vi "Dispensaor de Snacks.vi"() -> ()   [LabVIEW 2021]
panel:
  in  "Ring":u16(ring)
  out "Enum":T1(ring)
  in  "Dinero":i16
  in  "Tab Control":enum32{"Dispensador", "Inventario"}(tab)
  in  "Panel Frontal":T2
  in  "Reset":bool
  in  "Dispensador":bool
  in  "Productos":T3
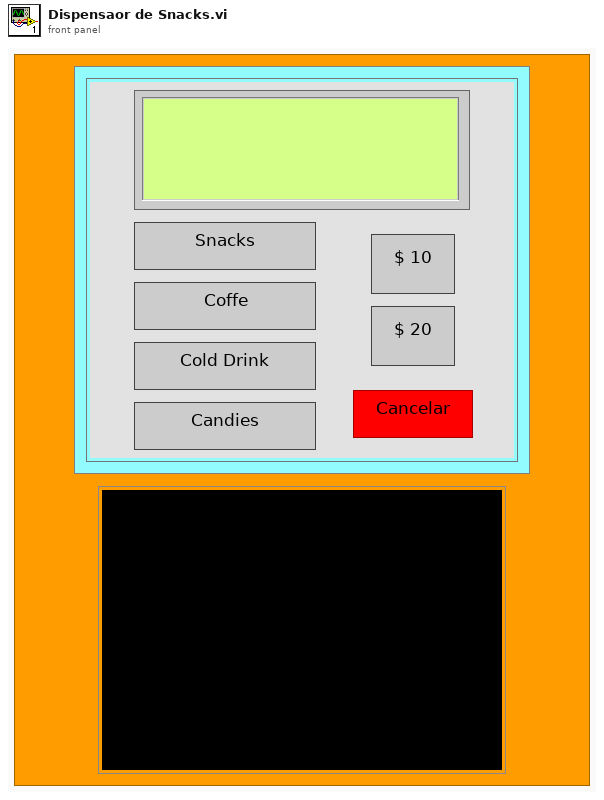
[diagram p1: front panel]
types:
  T1 = enum16{"Sin elegir", "Snacks", "Coffe", "Cold drink", "Candies"}
  T2 = cluster{"Snacks":bool, "Coffe":bool, "Cold drink":bool, "Candies":bool, "$ 10":bool, "$ 20":bool, "Cancelar":bool, "Pantalla":string, "Inventario":bool}
  T3 = cluster{"Snacks":i16, "Coffe":i16, "Cold drink":i16, "Candies":i16}
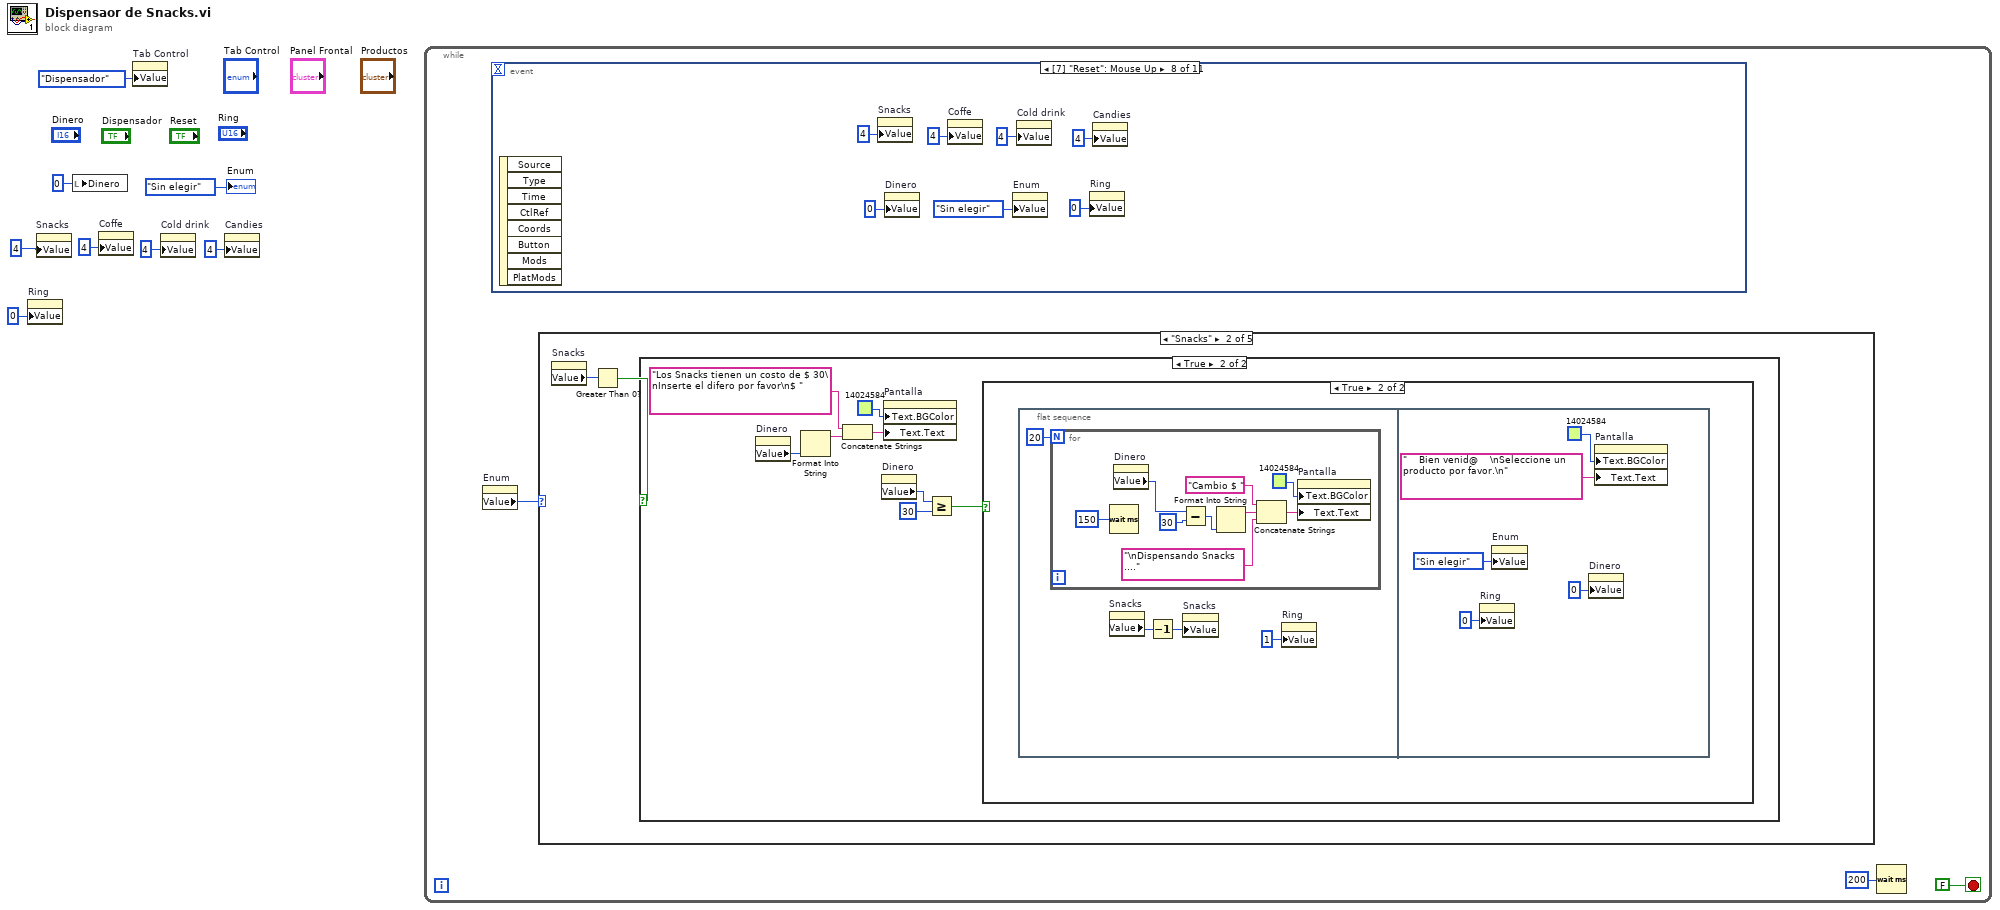
[diagram p0: block diagram]
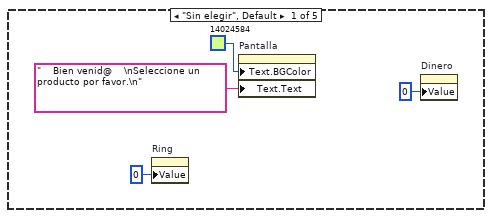
[diagram p2: hidden frame]
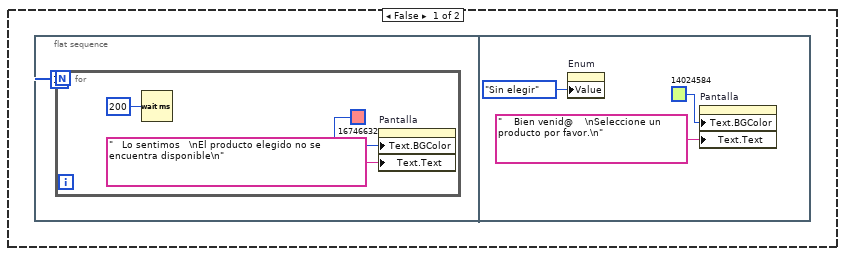
[diagram p3: hidden frame]
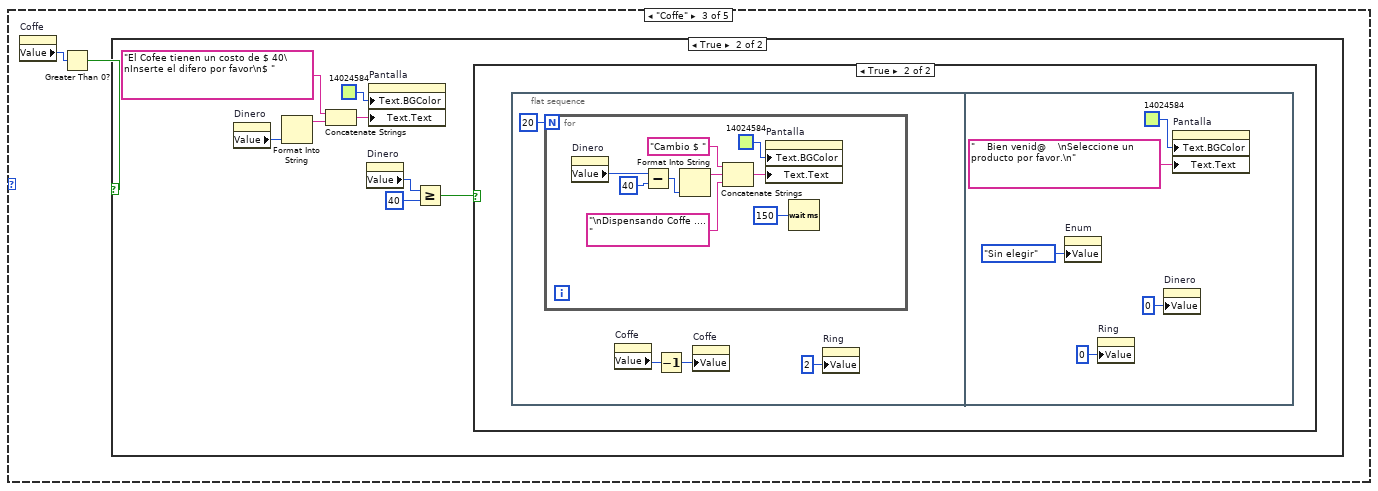
[diagram p5: hidden frame]
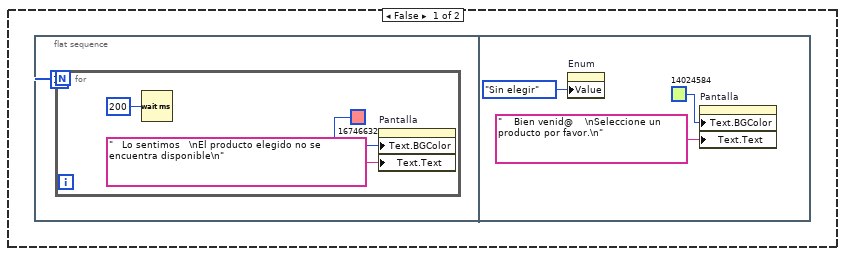
[diagram p6: hidden frame]
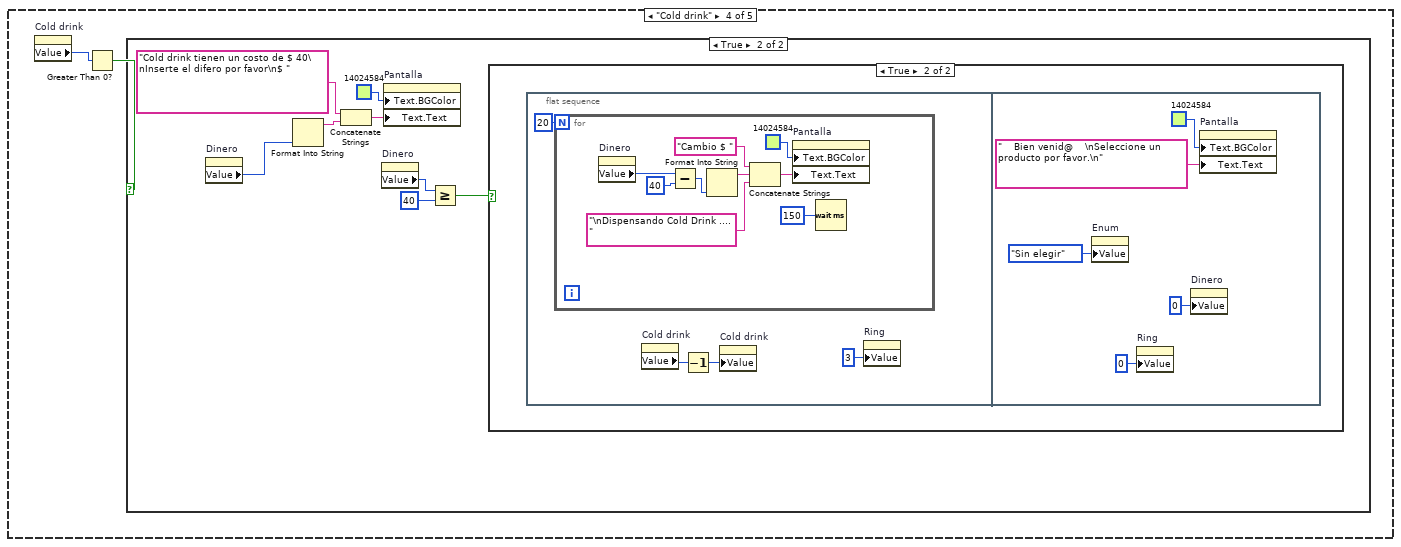
[diagram p8: hidden frame]
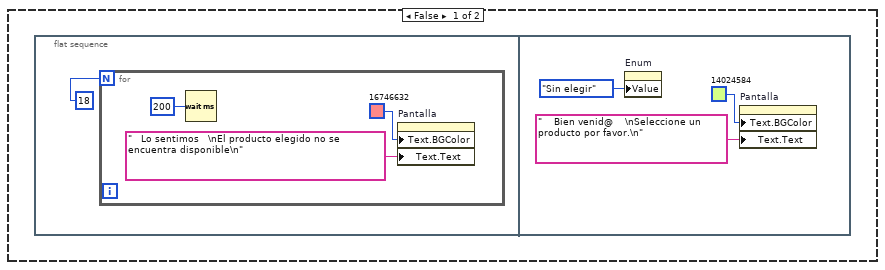
[diagram p9: hidden frame]
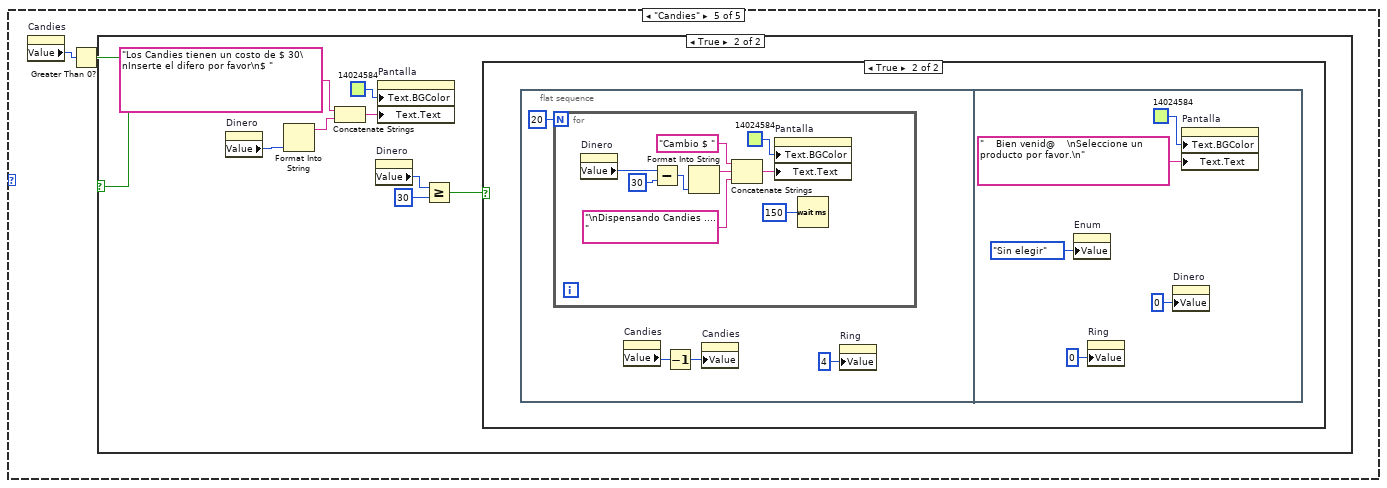
[diagram p11: hidden frame]
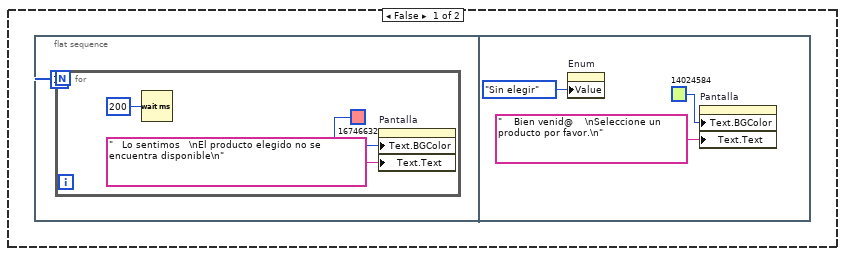
[diagram p12: hidden frame]
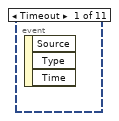
[diagram p14: hidden frame]
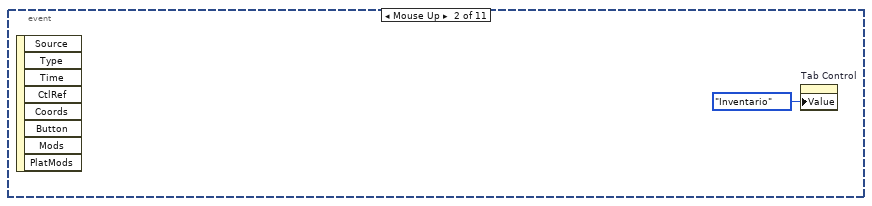
[diagram p15: hidden frame]
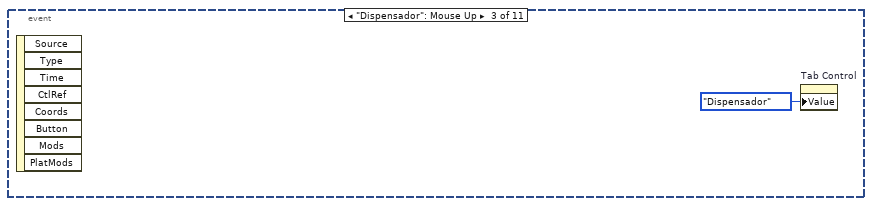
[diagram p16: hidden frame]
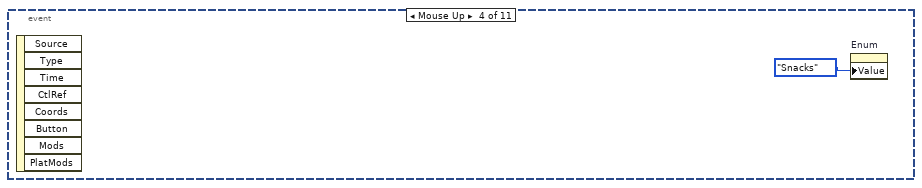
[diagram p17: hidden frame]
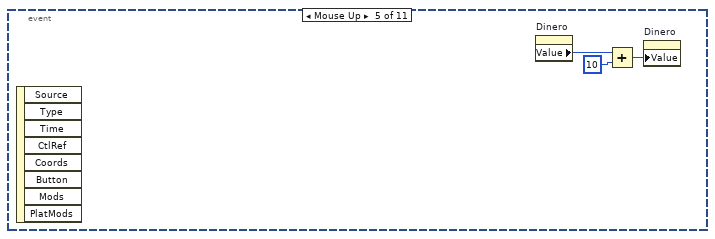
[diagram p18: hidden frame]
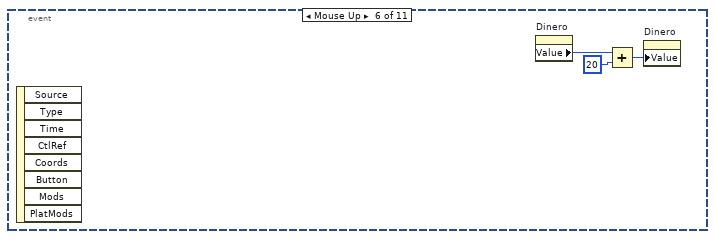
[diagram p19: hidden frame]
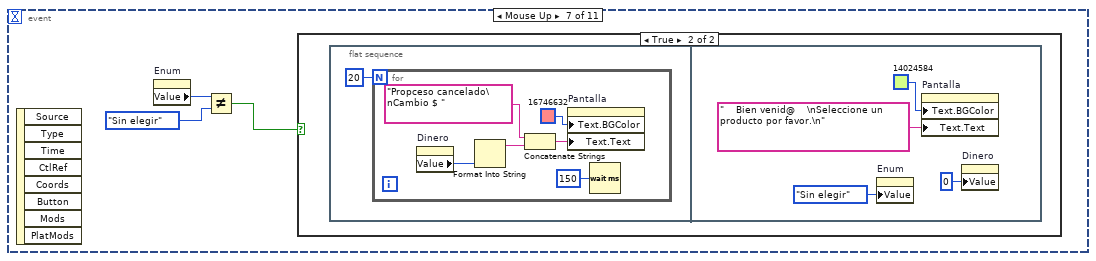
[diagram p20: hidden frame]
diagram:
  n1 = property on="Ring" class="Ring (strict)"("Value"=u16 0 ("Ring")) -> ()  [unwired: 2 in, 2 out]
  n2 = property on="Snacks" class="DigNum (strict)"("Value"=i16 4) -> ()  [unwired: 2 in, 2 out]
  n3 = local write "Dinero"(i16 0 ("Dinero")) -> ()
  n4 = property on="Coffe" class="DigNum (strict)"("Value"=i16 4) -> ()  [unwired: 2 in, 2 out]
  n5 = property on="Tab Control" class="TabCtl (strict)"("Value"=enum32{"Dispensador", "Inventario"}."Dispensador" ("Tab Control")) -> ()  [unwired: 2 in, 2 out]
  n6 = property on="Cold drink" class="DigNum (strict)"("Value"=i16 4) -> ()  [unwired: 2 in, 2 out]
  n7 = property on="Candies" class="DigNum (strict)"("Value"=i16 4) -> ()  [unwired: 2 in, 2 out]
  n8 = while {
    stop <- FALSE stop-if-true
    n9 = property on="Enum" class="Enum (strict)"() -> ("Value"=w9:T1)  [unwired: 2 in, 2 out]
    n10 = event shown="[7] \"Reset\": Mouse Up" {
      selector: _ -> [_ _ _ _ _ _ _ _ _ _ _]
      dyn-events: _ -> [_ _ _ _ _ _ _ _ _ _ _]
      timeout: _ -> [_ _ _ _ _ _ _ _ _ _ _]
      event Timeout {
        n11 = event-data() -> ()  [unwired: 1 in, 3 out]
      }
      event "Panel Frontal.Inventario": Mouse Up {
        n12 = event-data() -> ()  [unwired: 1 in, 8 out]
        n13 = property on="Tab Control" class="TabCtl (strict)"("Value"=enum32{"Dispensador", "Inventario"}."Inventario" ("Tab Control")) -> ()  [unwired: 2 in, 2 out]
      }
      event "Dispensador": Mouse Up {
        n14 = event-data() -> ()  [unwired: 1 in, 8 out]
        n15 = property on="Tab Control" class="TabCtl (strict)"("Value"=enum32{"Dispensador", "Inventario"}."Dispensador" ("Tab Control")) -> ()  [unwired: 2 in, 2 out]
      }
      event "Panel Frontal.Snacks": Mouse Up {
        n16 = event-data() -> ()  [unwired: 1 in, 8 out]
        n17 = property on="Enum" class="Enum (strict)"("Value"=T1."Snacks" ("Enum")) -> ()  [unwired: 2 in, 2 out]
      }
      event "Panel Frontal.$ 10": Mouse Up {
        n18 = event-data() -> ()  [unwired: 1 in, 8 out]
        n19 = property on="Dinero" class="DigNum (strict)"() -> ("Value"=w161:i16)  [unwired: 2 in, 2 out]
        n20 = Add(x=w161, y=i16 10) -> (x+y=w159:i16)
        n21 = property on="Dinero" class="DigNum (strict)"("Value"=w159) -> ()  [unwired: 2 in, 2 out]
      }
      event "Panel Frontal.$ 20": Mouse Up {
        n22 = event-data() -> ()  [unwired: 1 in, 8 out]
        n23 = property on="Dinero" class="DigNum (strict)"() -> ("Value"=w164:i16)  [unwired: 2 in, 2 out]
        n24 = Add(x=w164, y=i16 20) -> (x+y=w162:i16)
        n25 = property on="Dinero" class="DigNum (strict)"("Value"=w162) -> ()  [unwired: 2 in, 2 out]
      }
      event "Panel Frontal.Cancelar": Mouse Up {
        n26 = event-data() -> ()  [unwired: 1 in, 8 out]
        n27 = property on="Enum" class="Enum (strict)"() -> ("Value"=w167:T1)  [unwired: 2 in, 2 out]
        n28 = Not Equal?(x=w167, y=T1."Sin elegir") -> (x != y?=w165:bool)
        n29 = case shown="True" w165 {
          frame False {
          }
          frame True {
            n30 = flat-sequence {
              frame #0 {
                n31 = for {
                  N: 20 -> [_]
                  n32 = property on="Dinero" class="DigNum (strict)"() -> ("Value"=w173:i16)  [unwired: 2 in, 2 out]
                  n33 = Format Into String(w173) -> (resulting string=w171:string)  [unwired: 3 in, 1 out]
                  n34 = Concatenate Strings("Propceso cancelado\nCambio $ " ("Text.Text"), w171) -> (w170:string)
                  n35 = property on="Pantalla" class="Str"("Text.BGColor"=u32 16746632 ("Text.Text Colors:BG Color"), "Text.Text"=w170) -> ()  [unwired: 2 in, 2 out]
                  n36 = Wait (ms)(milliseconds to wait=u32 150) -> ()  [unwired: 1 out]
                }
              }
              frame #1 {
                n37 = property on="Enum" class="Enum (strict)"("Value"=T1."Sin elegir" ("Enum")) -> ()  [unwired: 2 in, 2 out]
                n38 = property on="Pantalla" class="Str"("Text.BGColor"=u32 14024584 ("Text.Text Colors:BG Color"), "Text.Text"="　 Bien venid@ 　\nSeleccione un producto por favor.\n") -> ()  [unwired: 2 in, 2 out]
                n39 = property on="Dinero" class="DigNum (strict)"("Value"=i16 0 ("Dinero")) -> ()  [unwired: 2 in, 2 out]
              }
            }
          }
        }
      }
      event "Reset": Mouse Up {
        n40 = event-data() -> ()  [unwired: 1 in, 8 out]
        n41 = property on="Snacks" class="DigNum (strict)"("Value"=i16 4) -> ()  [unwired: 2 in, 2 out]
        n42 = property on="Dinero" class="DigNum (strict)"("Value"=i16 0 ("Dinero")) -> ()  [unwired: 2 in, 2 out]
        n43 = property on="Coffe" class="DigNum (strict)"("Value"=i16 4) -> ()  [unwired: 2 in, 2 out]
        n44 = property on="Enum" class="Enum (strict)"("Value"=T1."Sin elegir" ("Enum")) -> ()  [unwired: 2 in, 2 out]
        n45 = property on="Cold drink" class="DigNum (strict)"("Value"=i16 4) -> ()  [unwired: 2 in, 2 out]
        n46 = property on="Ring" class="Ring (strict)"("Value"=u16 0 ("Ring")) -> ()  [unwired: 2 in, 2 out]
        n47 = property on="Candies" class="DigNum (strict)"("Value"=i16 4) -> ()  [unwired: 2 in, 2 out]
      }
      event "Panel Frontal.Cold drink": Mouse Up {
        n48 = event-data() -> ()  [unwired: 1 in, 8 out]
        n49 = property on="Enum" class="Enum (strict)"("Value"=T1."Cold drink" ("Enum")) -> ()  [unwired: 2 in, 2 out]
      }
      event "Panel Frontal.Candies": Mouse Up {
        n50 = event-data() -> ()  [unwired: 1 in, 8 out]
        n51 = property on="Enum" class="Enum (strict)"("Value"=T1."Candies" ("Enum")) -> ()  [unwired: 2 in, 2 out]
      }
      event "Panel Frontal.Coffe": Mouse Up {
        n52 = event-data() -> ()  [unwired: 1 in, 8 out]
        n53 = property on="Enum" class="Enum (strict)"("Value"=T1."Coffe" ("Enum")) -> ()  [unwired: 2 in, 2 out]
      }
    }
    n54 = case shown="\"Snacks\"" w9 {
      frame "Sin elegir", Default {
        n55 = property on="Ring" class="Ring (strict)"("Value"=u16 0 ("Ring")) -> ()  [unwired: 2 in, 2 out]
        n56 = property on="Pantalla" class="Str"("Text.BGColor"=u32 14024584 ("Text.Text Colors:BG Color"), "Text.Text"="　 Bien venid@ 　\nSeleccione un producto por favor.\n") -> ()  [unwired: 2 in, 2 out]
        n57 = property on="Dinero" class="DigNum (strict)"("Value"=i16 0 ("Dinero")) -> ()  [unwired: 2 in, 2 out]
      }
      frame "Snacks" {
        n58 = property on="Snacks" class="DigNum (strict)"() -> ("Value"=w17:i16)  [unwired: 2 in, 2 out]
        n59 = Greater Than 0?(x=w17) -> (x > 0?=w16:bool)
        n60 = case shown="True" w16 {
          frame False {
            n61 = flat-sequence {
              frame #0 {
                n62 = for {
                  N: 18 -> [_]
                  n63 = Wait (ms)(milliseconds to wait=u32 200) -> ()  [unwired: 1 out]
                  n64 = property on="Pantalla" class="Str"("Text.BGColor"=u32 16746632 ("Text.Text Colors:BG Color"), "Text.Text"="　Lo sentimos　\nEl producto elegido no se encuentra disponible\n") -> ()  [unwired: 2 in, 2 out]
                }
              }
              frame #1 {
                n65 = property on="Enum" class="Enum (strict)"("Value"=T1."Sin elegir" ("Enum")) -> ()  [unwired: 2 in, 2 out]
                n66 = property on="Pantalla" class="Str"("Text.BGColor"=u32 14024584 ("Text.Text Colors:BG Color"), "Text.Text"="　 Bien venid@ 　\nSeleccione un producto por favor.\n") -> ()  [unwired: 2 in, 2 out]
              }
            }
          }
          frame True {
            n67 = property on="Dinero" class="DigNum (strict)"() -> ("Value"=w31:i16)  [unwired: 2 in, 2 out]
            n68 = Format Into String(w31) -> (resulting string=w29:string)  [unwired: 3 in, 1 out]
            n69 = Concatenate Strings("Los Snacks tienen un costo de $ 30\nInserte el difero por favor\n$ " ("Text.Text"), w29) -> (w28:string)
            n70 = property on="Dinero" class="DigNum (strict)"() -> ("Value"=w27:i16)  [unwired: 2 in, 2 out]
            n71 = property on="Pantalla" class="Str"("Text.BGColor"=u32 14024584 ("Text.Text Colors:BG Color"), "Text.Text"=w28) -> ()  [unwired: 2 in, 2 out]
            n72 = Greater Or Equal?(x=w27, y=i16 30) -> (x >= y?=w25:bool)
            n73 = case shown="True" w25 {
              frame False {
              }
              frame True {
                n74 = flat-sequence {
                  frame #0 {
                    n75 = for {
                      N: 20 -> [_]
                      n76 = Wait (ms)(milliseconds to wait=u32 150) -> ()  [unwired: 1 out]
                      n77 = property on="Dinero" class="DigNum (strict)"() -> ("Value"=w44:i16)  [unwired: 2 in, 2 out]
                      n78 = Subtract(x=w44, y=i16 30) -> (x-y=w42:i16)
                      n79 = Format Into String(w42) -> (resulting string=w40:string)  [unwired: 3 in, 1 out]
                      n80 = Concatenate Strings("Cambio $ " ("string"), w40, "\nDispensando Snacks ...." ("string")) -> (w38:string)
                      n81 = property on="Pantalla" class="Str"("Text.BGColor"=u32 14024584 ("Text.Text Colors:BG Color"), "Text.Text"=w38) -> ()  [unwired: 2 in, 2 out]
                    }
                    n82 = property on="Snacks" class="DigNum (strict)"() -> ("Value"=w34:i16)  [unwired: 2 in, 2 out]
                    n83 = Decrement(x=w34) -> (x-1=w35:i16)
                    n84 = property on="Snacks" class="DigNum (strict)"("Value"=w35) -> ()  [unwired: 2 in, 2 out]
                    n85 = property on="Ring" class="Ring (strict)"("Value"=u16 1 ("Ring")) -> ()  [unwired: 2 in, 2 out]
                  }
                  frame #1 {
                    n86 = property on="Ring" class="Ring (strict)"("Value"=u16 0 ("Ring")) -> ()  [unwired: 2 in, 2 out]
                    n87 = property on="Enum" class="Enum (strict)"("Value"=T1."Sin elegir" ("Enum")) -> ()  [unwired: 2 in, 2 out]
                    n88 = property on="Dinero" class="DigNum (strict)"("Value"=i16 0 ("Dinero")) -> ()  [unwired: 2 in, 2 out]
                    n89 = property on="Pantalla" class="Str"("Text.BGColor"=u32 14024584 ("Text.Text Colors:BG Color"), "Text.Text"="　 Bien venid@ 　\nSeleccione un producto por favor.\n") -> ()  [unwired: 2 in, 2 out]
                  }
                }
              }
            }
          }
        }
      }
      frame "Coffe" {
        n90 = property on="Coffe" class="DigNum (strict)"() -> ("Value"=w52:i16)  [unwired: 2 in, 2 out]
        n91 = Greater Than 0?(x=w52) -> (x > 0?=w51:bool)
        n92 = case shown="True" w51 {
          frame False {
            n93 = flat-sequence {
              frame #0 {
                n94 = for {
                  N: 18 -> [_]
                  n95 = Wait (ms)(milliseconds to wait=u32 200) -> ()  [unwired: 1 out]
                  n96 = property on="Pantalla" class="Str"("Text.BGColor"=u32 16746632 ("Text.Text Colors:BG Color"), "Text.Text"="　Lo sentimos　\nEl producto elegido no se encuentra disponible\n") -> ()  [unwired: 2 in, 2 out]
                }
              }
              frame #1 {
                n97 = property on="Enum" class="Enum (strict)"("Value"=T1."Sin elegir" ("Enum")) -> ()  [unwired: 2 in, 2 out]
                n98 = property on="Pantalla" class="Str"("Text.BGColor"=u32 14024584 ("Text.Text Colors:BG Color"), "Text.Text"="　 Bien venid@ 　\nSeleccione un producto por favor.\n") -> ()  [unwired: 2 in, 2 out]
              }
            }
          }
          frame True {
            n99 = property on="Dinero" class="DigNum (strict)"() -> ("Value"=w66:i16)  [unwired: 2 in, 2 out]
            n100 = Format Into String(w66) -> (resulting string=w64:string)  [unwired: 3 in, 1 out]
            n101 = Concatenate Strings("El Cofee tienen un costo de $ 40\nInserte el difero por favor\n$ " ("Text.Text"), w64) -> (w63:string)
            n102 = property on="Dinero" class="DigNum (strict)"() -> ("Value"=w62:i16)  [unwired: 2 in, 2 out]
            n103 = property on="Pantalla" class="Str"("Text.BGColor"=u32 14024584 ("Text.Text Colors:BG Color"), "Text.Text"=w63) -> ()  [unwired: 2 in, 2 out]
            n104 = Greater Or Equal?(x=w62, y=i16 40) -> (x >= y?=w60:bool)
            n105 = case shown="True" w60 {
              frame False {
              }
              frame True {
                n106 = flat-sequence {
                  frame #0 {
                    n107 = for {
                      N: 20 -> [_]
                      n108 = property on="Dinero" class="DigNum (strict)"() -> ("Value"=w79:i16)  [unwired: 2 in, 2 out]
                      n109 = Subtract(x=w79, y=i16 40) -> (x-y=w77:i16)
                      n110 = Format Into String(w77) -> (resulting string=w75:string)  [unwired: 3 in, 1 out]
                      n111 = Concatenate Strings("Cambio $ " ("string"), w75, "\nDispensando Coffe ...." ("string")) -> (w73:string)
                      n112 = property on="Pantalla" class="Str"("Text.BGColor"=u32 14024584 ("Text.Text Colors:BG Color"), "Text.Text"=w73) -> ()  [unwired: 2 in, 2 out]
                      n113 = Wait (ms)(milliseconds to wait=u32 150) -> ()  [unwired: 1 out]
                    }
                    n114 = property on="Coffe" class="DigNum (strict)"() -> ("Value"=w69:i16)  [unwired: 2 in, 2 out]
                    n115 = Decrement(x=w69) -> (x-1=w70:i16)
                    n116 = property on="Coffe" class="DigNum (strict)"("Value"=w70) -> ()  [unwired: 2 in, 2 out]
                    n117 = property on="Ring" class="Ring (strict)"("Value"=u16 2 ("Ring")) -> ()  [unwired: 2 in, 2 out]
                  }
                  frame #1 {
                    n118 = property on="Enum" class="Enum (strict)"("Value"=T1."Sin elegir" ("Enum")) -> ()  [unwired: 2 in, 2 out]
                    n119 = property on="Ring" class="Ring (strict)"("Value"=u16 0 ("Ring")) -> ()  [unwired: 2 in, 2 out]
                    n120 = property on="Dinero" class="DigNum (strict)"("Value"=i16 0 ("Dinero")) -> ()  [unwired: 2 in, 2 out]
                    n121 = property on="Pantalla" class="Str"("Text.BGColor"=u32 14024584 ("Text.Text Colors:BG Color"), "Text.Text"="　 Bien venid@ 　\nSeleccione un producto por favor.\n") -> ()  [unwired: 2 in, 2 out]
                  }
                }
              }
            }
          }
        }
      }
      frame "Cold drink" {
        n122 = property on="Cold drink" class="DigNum (strict)"() -> ("Value"=w86:i16)  [unwired: 2 in, 2 out]
        n123 = Greater Than 0?(x=w86) -> (x > 0?=w87:bool)
        n124 = case shown="True" w87 {
          frame False {
            n125 = flat-sequence {
              frame #0 {
                n126 = for {
                  N: 18 -> [_]
                  n127 = Wait (ms)(milliseconds to wait=u32 200) -> ()  [unwired: 1 out]
                  n128 = property on="Pantalla" class="Str"("Text.BGColor"=u32 16746632 ("Text.Text Colors:BG Color"), "Text.Text"="　Lo sentimos　\nEl producto elegido no se encuentra disponible\n") -> ()  [unwired: 2 in, 2 out]
                }
              }
              frame #1 {
                n129 = property on="Enum" class="Enum (strict)"("Value"=T1."Sin elegir" ("Enum")) -> ()  [unwired: 2 in, 2 out]
                n130 = property on="Pantalla" class="Str"("Text.BGColor"=u32 14024584 ("Text.Text Colors:BG Color"), "Text.Text"="　 Bien venid@ 　\nSeleccione un producto por favor.\n") -> ()  [unwired: 2 in, 2 out]
              }
            }
          }
          frame True {
            n131 = property on="Dinero" class="DigNum (strict)"() -> ("Value"=w101:i16)  [unwired: 2 in, 2 out]
            n132 = Format Into String(w101) -> (resulting string=w99:string)  [unwired: 3 in, 1 out]
            n133 = Concatenate Strings("Cold drink tienen un costo de $ 40\nInserte el difero por favor\n$ " ("Text.Text"), w99) -> (w98:string)
            n134 = property on="Dinero" class="DigNum (strict)"() -> ("Value"=w97:i16)  [unwired: 2 in, 2 out]
            n135 = property on="Pantalla" class="Str"("Text.BGColor"=u32 14024584 ("Text.Text Colors:BG Color"), "Text.Text"=w98) -> ()  [unwired: 2 in, 2 out]
            n136 = Greater Or Equal?(x=w97, y=i16 40) -> (x >= y?=w95:bool)
            n137 = case shown="True" w95 {
              frame False {
              }
              frame True {
                n138 = flat-sequence {
                  frame #0 {
                    n139 = for {
                      N: 20 -> [_]
                      n140 = property on="Dinero" class="DigNum (strict)"() -> ("Value"=w114:i16)  [unwired: 2 in, 2 out]
                      n141 = Subtract(x=w114, y=i16 40) -> (x-y=w112:i16)
                      n142 = Format Into String(w112) -> (resulting string=w110:string)  [unwired: 3 in, 1 out]
                      n143 = Concatenate Strings("Cambio $ " ("string"), w110, "\nDispensando Cold Drink ...." ("string")) -> (w108:string)
                      n144 = property on="Pantalla" class="Str"("Text.BGColor"=u32 14024584 ("Text.Text Colors:BG Color"), "Text.Text"=w108) -> ()  [unwired: 2 in, 2 out]
                      n145 = Wait (ms)(milliseconds to wait=u32 150) -> ()  [unwired: 1 out]
                    }
                    n146 = property on="Cold drink" class="DigNum (strict)"() -> ("Value"=w104:i16)  [unwired: 2 in, 2 out]
                    n147 = Decrement(x=w104) -> (x-1=w105:i16)
                    n148 = property on="Cold drink" class="DigNum (strict)"("Value"=w105) -> ()  [unwired: 2 in, 2 out]
                    n149 = property on="Ring" class="Ring (strict)"("Value"=u16 3 ("Ring")) -> ()  [unwired: 2 in, 2 out]
                  }
                  frame #1 {
                    n150 = property on="Enum" class="Enum (strict)"("Value"=T1."Sin elegir" ("Enum")) -> ()  [unwired: 2 in, 2 out]
                    n151 = property on="Ring" class="Ring (strict)"("Value"=u16 0 ("Ring")) -> ()  [unwired: 2 in, 2 out]
                    n152 = property on="Dinero" class="DigNum (strict)"("Value"=i16 0 ("Dinero")) -> ()  [unwired: 2 in, 2 out]
                    n153 = property on="Pantalla" class="Str"("Text.BGColor"=u32 14024584 ("Text.Text Colors:BG Color"), "Text.Text"="　 Bien venid@ 　\nSeleccione un producto por favor.\n") -> ()  [unwired: 2 in, 2 out]
                  }
                }
              }
            }
          }
        }
      }
      frame "Candies" {
        n154 = property on="Candies" class="DigNum (strict)"() -> ("Value"=w122:i16)  [unwired: 2 in, 2 out]
        n155 = Greater Than 0?(x=w122) -> (x > 0?=w121:bool)
        n156 = case shown="True" w121 {
          frame False {
            n157 = flat-sequence {
              frame #0 {
                n158 = for {
                  N: 18 -> [_]
                  n159 = Wait (ms)(milliseconds to wait=u32 200) -> ()  [unwired: 1 out]
                  n160 = property on="Pantalla" class="Str"("Text.BGColor"=u32 16746632 ("Text.Text Colors:BG Color"), "Text.Text"="　Lo sentimos　\nEl producto elegido no se encuentra disponible\n") -> ()  [unwired: 2 in, 2 out]
                }
              }
              frame #1 {
                n161 = property on="Enum" class="Enum (strict)"("Value"=T1."Sin elegir" ("Enum")) -> ()  [unwired: 2 in, 2 out]
                n162 = property on="Pantalla" class="Str"("Text.BGColor"=u32 14024584 ("Text.Text Colors:BG Color"), "Text.Text"="　 Bien venid@ 　\nSeleccione un producto por favor.\n") -> ()  [unwired: 2 in, 2 out]
              }
            }
          }
          frame True {
            n163 = property on="Dinero" class="DigNum (strict)"() -> ("Value"=w136:i16)  [unwired: 2 in, 2 out]
            n164 = Format Into String(w136) -> (resulting string=w134:string)  [unwired: 3 in, 1 out]
            n165 = Concatenate Strings("Los Candies tienen un costo de $ 30\nInserte el difero por favor\n$ " ("Text.Text"), w134) -> (w133:string)
            n166 = property on="Dinero" class="DigNum (strict)"() -> ("Value"=w132:i16)  [unwired: 2 in, 2 out]
            n167 = property on="Pantalla" class="Str"("Text.BGColor"=u32 14024584 ("Text.Text Colors:BG Color"), "Text.Text"=w133) -> ()  [unwired: 2 in, 2 out]
            n168 = Greater Or Equal?(x=w132, y=i16 30) -> (x >= y?=w130:bool)
            n169 = case shown="True" w130 {
              frame False {
              }
              frame True {
                n170 = flat-sequence {
                  frame #0 {
                    n171 = for {
                      N: 20 -> [_]
                      n172 = property on="Dinero" class="DigNum (strict)"() -> ("Value"=w149:i16)  [unwired: 2 in, 2 out]
                      n173 = Subtract(x=w149, y=i16 30) -> (x-y=w147:i16)
                      n174 = Format Into String(w147) -> (resulting string=w145:string)  [unwired: 3 in, 1 out]
                      n175 = Concatenate Strings("Cambio $ " ("string"), w145, "\nDispensando Candies ...." ("string")) -> (w143:string)
                      n176 = property on="Pantalla" class="Str"("Text.BGColor"=u32 14024584 ("Text.Text Colors:BG Color"), "Text.Text"=w143) -> ()  [unwired: 2 in, 2 out]
                      n177 = Wait (ms)(milliseconds to wait=u32 150) -> ()  [unwired: 1 out]
                    }
                    n178 = property on="Candies" class="DigNum (strict)"() -> ("Value"=w139:i16)  [unwired: 2 in, 2 out]
                    n179 = Decrement(x=w139) -> (x-1=w140:i16)
                    n180 = property on="Candies" class="DigNum (strict)"("Value"=w140) -> ()  [unwired: 2 in, 2 out]
                    n181 = property on="Ring" class="Ring (strict)"("Value"=u16 4 ("Ring")) -> ()  [unwired: 2 in, 2 out]
                  }
                  frame #1 {
                    n182 = property on="Enum" class="Enum (strict)"("Value"=T1."Sin elegir" ("Enum")) -> ()  [unwired: 2 in, 2 out]
                    n183 = property on="Ring" class="Ring (strict)"("Value"=u16 0 ("Ring")) -> ()  [unwired: 2 in, 2 out]
                    n184 = property on="Dinero" class="DigNum (strict)"("Value"=i16 0 ("Dinero")) -> ()  [unwired: 2 in, 2 out]
                    n185 = property on="Pantalla" class="Str"("Text.BGColor"=u32 14024584 ("Text.Text Colors:BG Color"), "Text.Text"="　 Bien venid@ 　\nSeleccione un producto por favor.\n") -> ()  [unwired: 2 in, 2 out]
                  }
                }
              }
            }
          }
        }
      }
    }
    n186 = Wait (ms)(milliseconds to wait=u32 200) -> ()  [unwired: 1 out]
  }
  "Enum" <- T1."Sin elegir"
